vi "OpenReadWriteCloseTestClass4.vi"() -> ()   [LabVIEW 2013, in "EMV-Test.lvlib"]
uses:
  EMV-Test.lvlib
  classes/Devices/Class4/Class 4.lvclass
panel:
  in  "input":string
  out "Return String":string
  in  "VISA resource name":refnum<visa-resource-name>
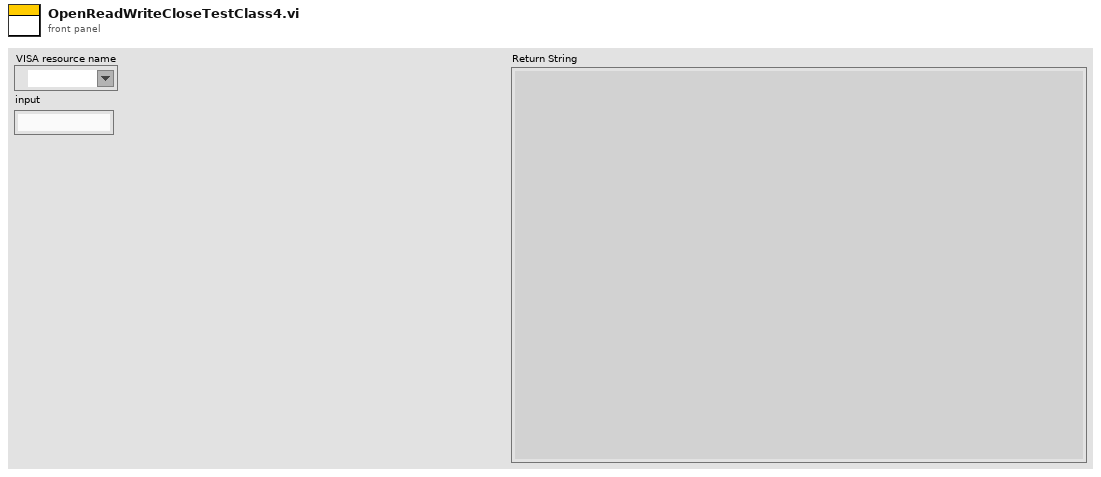
[diagram p1: front panel]
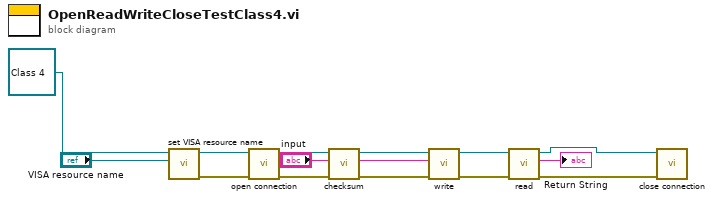
[diagram p0: block diagram]
diagram:
  n1 = call-dynamic "set VISA resource name.vi"("VISA resource name"="VISA resource name", "DeviceInterface (Eingang)"=refnum<class "Class 4.lvclass"> refnum ("Class 4.lvclass")) -> ("error out"=w13:errorcluster, "DeviceInterface (Ausgang)"=w14:refnum<class "Class 4.lvclass">)  [unwired: 8 in]
  n2 = call-dynamic "open connection.vi"("error in (no error)"=w13, "Class 4 Eingang"=w14) -> ("error out"=w11:errorcluster, "Class 4 Ausgang"=w12:refnum<class "Class 4.lvclass">)  [unwired: 8 in]
  n3 = call-dynamic "checksum.vi"("error in (no error)"=w11, "input"="input", "Class 4 in"=w12) -> ("error out"=w9:errorcluster, "output"=w8:string, "Class 4 out"=w10:refnum<class "Class 4.lvclass">)  [unwired: 6 in]
  n4 = call-dynamic "write.vi"("error in (no error)"=w9, "String to send"=w8, "Class 4 in"=w10) -> ("error out"=w6:errorcluster, "Class 4 out"=w7:refnum<class "Class 4.lvclass">)  [unwired: 7 in]
  n5 = call-dynamic "read.vi"("error in (no error)"=w6, "Class 4 in"=w7) -> ("error out"=w3:errorcluster, "Return String"=→"Return String":string, "Class 4 out"=w4:refnum<class "Class 4.lvclass">)  [unwired: 7 in]
  n6 = call-dynamic "close connection.vi"("error in (no error)"=w3, "Class 4 in"=w4) -> ()  [unwired: 8 in, 2 out]
